vi "myFriendthePelletIdentifier00Subtask3redo.vi"() -> ()   [LabVIEW 2016]
uses:
  <vilib>/NXT/Block Support/NXT_InputPort.ctl
  <vilib>/NXT/Dual Mode Library/Waits/Wait_Bump.vi
  <vilib>/NXT/Dual Mode Library/Sensors/Touch_Pressed.vi
  <vilib>/NXT/Dual Mode Library/Sensors/EV3_Color_RGB.vi
  <vilib>/NXT/Dual Mode Library/prims/inRangeAndCoerce/inRangeAndCoerce_int.vi
  <vilib>/NXT/Dual Mode Library/Sensors/EV3_Color_Color.vi
panel:
  out "Color Size\n  Output 9":string
  out "Color Size\n  Output 8":string
  out "Color Size\n  Output 7":string
  out "Color Size\n  Output":string
  out "Color Size\n  Output 6":string
  out "Color Size\n  Output 4":string
  out "Color Size\n  Output 3":string
  out "Color Size\n  Output 2":string
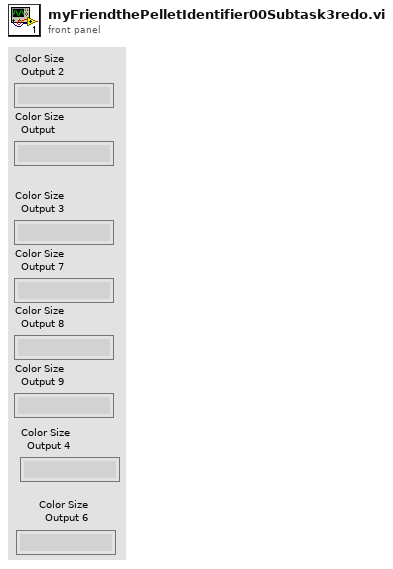
[diagram p1: front panel]
types:
  T1 = typedef "NXT_InputPort.ctl" = u32
  T2 = typedef "LVHSConnector.ctl" = refnum<class "BrickReference.lvclass">
  T3 = typedef "ColorSensorColors.ctl" = enum16{"No Color", "Black", "Blue", "Green", "Yellow", "Red", "White", "Brown"}
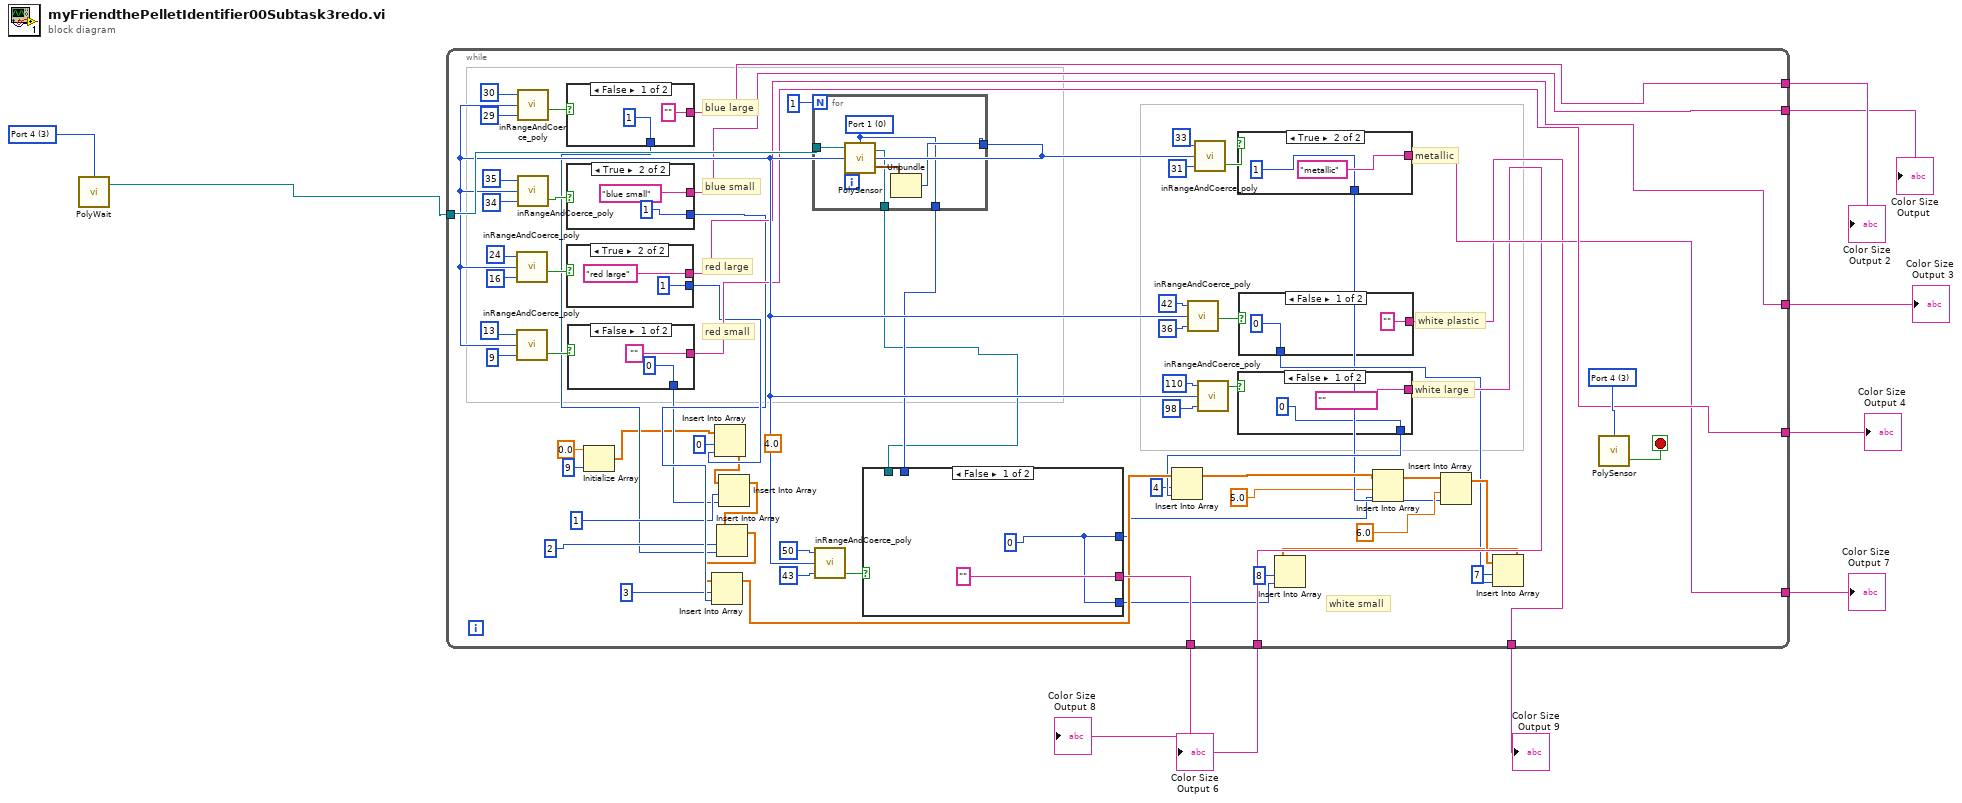
[diagram p0: block diagram]
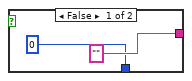
[diagram p2: hidden frame]
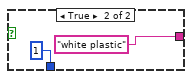
[diagram p3: hidden frame]
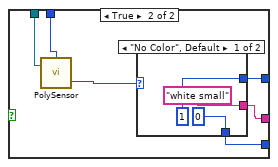
[diagram p4: hidden frame]
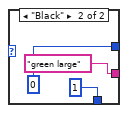
[diagram p5: hidden frame]
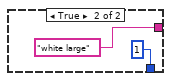
[diagram p6: hidden frame]
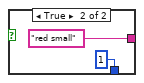
[diagram p7: hidden frame]
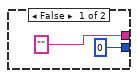
[diagram p8: hidden frame]
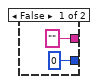
[diagram p9: hidden frame]
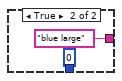
[diagram p10: hidden frame]
diagram:
  w9 = T1 3 items=["Port 1", "Port 2", "Port 3", "Port 4"] ("Port (Port 1)")
  n1 = call-poly <vilib>:"PolyWait.vi"("Port (Port 1)"=w9) -> ("NXT/EV3"=w10:T2)  [unwired: 3 in]
  n2 = while {
    tunnel: w10 -> [w54]
    tunnel: [w48] -> w8
    tunnel: [w47] -> w7
    tunnel: [w46] -> w6
    tunnel: [w45] -> w5
    tunnel: [w44] -> w4
    tunnel: [w43] -> w3
    tunnel: [w42] -> w2
    tunnel: [w41] -> w1
    stop <- w57 stop-if-true
    (unwired) sgl 4.0 ("Time (1 sec)")
    w56 = T1 3 items=["Port 1", "Port 2", "Port 3", "Port 4"] ("Port (Port 1)")
    # "metallic"
    # "white plastic"
    # "white small"
    # "white large"
    # "red small"
    # "red large"
    # "blue small"
    # "blue large"
    n3 = Initialize Array(0.0 ("element"), 9 ("dimension size")) -> (w29:dbl[])
    n4 = for {
      N: 1 -> [_]
      tunnel: w54 -> [w82]
      tunnel: [w81] -> w50
      tunnel: [w80] -> w40
      tunnel: [w79] -> w49
      w79 = T1 0 items=["Port 1", "Port 2", "Port 3", "Port 4"] ("Port (Port 1)")
      n5 = call-poly <vilib>:"PolySensor.vi"("NXT/EV3"=w82, "Port (Port 1)"=w79) -> ("RGB Color"=w83:cluster{"Red":u8, "Green":u8, "Blue":u8}, "NXT/EV3"=w80:T2)  [unwired: 1 in]
      n6 = Unbundle(w83) -> ("Green"=w81:u8)  [unwired: 2 out]
    }
    n7 = call-poly <vilib>:"inRangeAndCoerce_poly.vi"("lower limit"=16, "x"=w50, "upper limit"=24) -> ("In Range?"=w63:bool)  [unwired: 1 out]
    n8 = call-poly <vilib>:"inRangeAndCoerce_poly.vi"("lower limit"=9, "x"=w50, "upper limit"=13) -> ("In Range?"=w62:bool)  [unwired: 1 out]
    n9 = call-poly <vilib>:"inRangeAndCoerce_poly.vi"("lower limit"=29, "x"=w50, "upper limit"=30) -> ("In Range?"=w65:bool)  [unwired: 1 out]
    n10 = call-poly <vilib>:"inRangeAndCoerce_poly.vi"("lower limit"=34, "x"=w50, "upper limit"=35) -> ("In Range?"=w64:bool)  [unwired: 1 out]
    n11 = case shown="False" w65 {
      tunnel: ["" "blue large"] -> w48
      tunnel: [1 0] -> w31
      frame False {
      }
      frame True {
      }
    }
    n12 = case shown="True" w64 {
      tunnel: ["" "blue small"] -> w47
      tunnel: [0 1] -> w35
      frame False {
      }
      frame True {
      }
    }
    n13 = case shown="True" w63 {
      tunnel: ["" "red large"] -> w46
      tunnel: [0 1] -> w36
      frame False {
      }
      frame True {
      }
    }
    n14 = case shown="False" w62 {
      tunnel: ["" "red small"] -> w45
      tunnel: [0 1] -> w30
      frame False {
      }
      frame True {
      }
    }
    n15 = Insert Into Array(array=w29, index=0, new element=w36) -> (w28:dbl[])
    n16 = Insert Into Array(array=w28, index=1, new element=w30) -> (w27:dbl[])
    n17 = Insert Into Array(array=w27, index=2, new element=w31) -> (w26:dbl[])
    n18 = Insert Into Array(array=w26, index=3, new element=w35) -> (w25:dbl[])
    n19 = call-poly <vilib>:"inRangeAndCoerce_poly.vi"("lower limit"=43, "x"=w50, "upper limit"=50) -> ("In Range?"=w60:bool)  [unwired: 1 out]
    n20 = case shown="False" w60 {
      tunnel: ["" w97] -> w42
      tunnel: w49 -> [_ w99]
      tunnel: w40 -> [_ w96]
      tunnel: [w92 w95] -> w12
      tunnel: [w92 w94] -> w19
      frame False {
        w92 = 0
      }
      frame True {
        n21 = call-poly <vilib>:"PolySensor.vi"("NXT/EV3"=w96, "Port (Port 1)"=w99) -> ("Detected Color"=w98:T3)  [unwired: 1 in, 1 out]
        n22 = case shown="\"No Color\", Default" w98 {
          tunnel: ["white small" "green large"] -> w97
          tunnel: [1 0] -> w95
          tunnel: [0 1] -> w94
          frame "No Color", Default {
          }
          frame "Black" {
          }
        }
      }
    }
    n23 = call-poly <vilib>:"inRangeAndCoerce_poly.vi"("lower limit"=36, "x"=w50, "upper limit"=42) -> ("In Range?"=w59:bool)  [unwired: 1 out]
    n24 = call-poly <vilib>:"inRangeAndCoerce_poly.vi"("lower limit"=31, "x"=w50, "upper limit"=33) -> ("In Range?"=w51:bool)  [unwired: 1 out]
    n25 = call-poly <vilib>:"inRangeAndCoerce_poly.vi"("lower limit"=98, "x"=w50, "upper limit"=110) -> ("In Range?"=w61:bool)  [unwired: 1 out]
    n26 = case shown="True" w51 {
      tunnel: ["" "metallic"] -> w44
      tunnel: [0 1] -> w13
      frame False {
      }
      frame True {
      }
    }
    n27 = case shown="False" w61 {
      tunnel: ["" "white large"] -> w41
      tunnel: [0 1] -> w21
      frame False {
      }
      frame True {
      }
    }
    n28 = Insert Into Array(array=w25, index=4, new element=w21) -> (w15:dbl[])
    n29 = case shown="False" w59 {
      tunnel: ["" "white plastic"] -> w43
      tunnel: [0 1] -> w18
      frame False {
      }
      frame True {
      }
    }
    n30 = Insert Into Array(array=w15, index=5.0 ("new element/subarray"), new element=w12) -> (w24:dbl[])
    n31 = Insert Into Array(array=w24, index=6.0 ("new element/subarray"), new element=w13) -> (w23:dbl[])
    n32 = Insert Into Array(array=w23, index=7, new element=w18) -> (w22:dbl[])
    n33 = Insert Into Array(array=w22, index=8, new element=w19) -> ()  [unwired: 1 out]
    n34 = call-poly <vilib>:"PolySensor.vi"("Port (Port 1)"=w56) -> ("Yes / No"=w57:bool)  [unwired: 2 in, 1 out]
  }
  "Color Size\n  Output 2" <- w8
  "Color Size\n  Output 3" <- w6
  "Color Size\n  Output" <- w7
  "Color Size\n  Output 9" <- w3
  "Color Size\n  Output 7" <- w4
  "Color Size\n  Output 4" <- w5
  "Color Size\n  Output 8" <- w2
  "Color Size\n  Output 6" <- w1
